vi "pulse_status.vi"(8 "error in":errorcluster) -> (0 "error out":errorcluster, 3 "status":string)   [LabVIEW 2013]
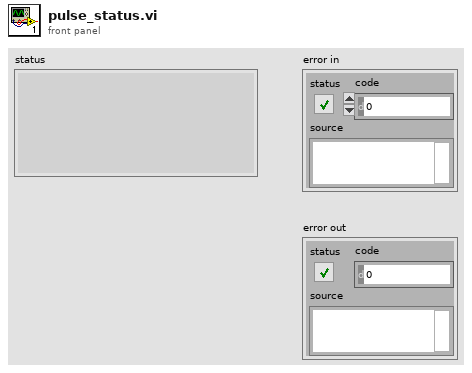
[diagram p1: front panel]
types:
  T1 = cluster{"high times":dbl, "low times":dbl, "pulse number":i32, "cmd":string, "status":string}
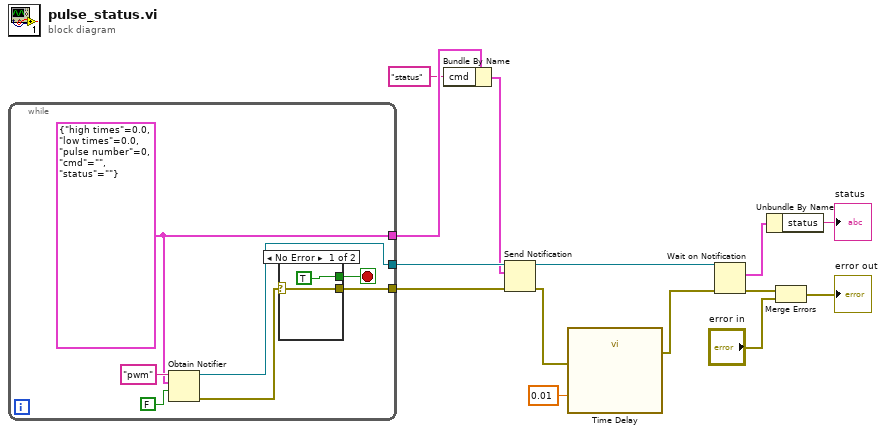
[diagram p0: block diagram]
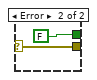
[diagram p2: hidden frame]
diagram:
  n1 = while {
    tunnel: [w19] -> w14
    tunnel: [w15] -> w13
    tunnel: [w18] -> w12
    stop <- w16 stop-if-true
    w18 = T1 {"high times"=0.0, "low times"=0.0, "pulse number"=0, "cmd"="", "status"=""}
    n2 = Obtain Notifier(name (unnamed)="pwm", notification data type=w18, create if not found? (T)=FALSE) -> (notifier out=w19:refnum<notifier>, error out=w17:errorcluster)  [unwired: 1 in, 1 out]
    n3 = case shown="No Error" w17 {
      selector: w17 -> [w22 w24]
      tunnel: [TRUE FALSE] -> w16
      tunnel: [w22 w24] -> w15
      frame No Error {
      }
      frame Error {
      }
    }
  }
  n4 = Bundle By Name(cluster=w12, "cmd"="status") -> (w10:T1)
  n5 = Send Notification(notification=w10, notifier=w14, error in (no error)=w13) -> (notifier out=w6:refnum<notifier>, error out=w3:errorcluster)
  n6 = call "Time Delay"("error in (no error)"=w3, "Delay Time (s)"=0.01) -> ("error out"=w2:errorcluster)  [unwired: 9 in]
  n7 = Wait on Notification(notifier=w6, error in (no error)=w2) -> (notification=w5:T1, error out=w7:errorcluster)  [unwired: 2 in, 2 out]
  n8 = Unbundle By Name(w5) -> ("status"=→"status":string)
  n9 = Merge Errors(w7, "error in") -> (→"error out":errorcluster)
